vi "piezoWriteStart.vi"   [LabVIEW 2017]
uses:
  globalDevices.vi
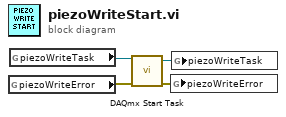
[diagram p0: block diagram]
diagram:
  n1 = global read "globalDevices.vi" "piezoWriteError"() -> (w3:errorcluster)
  n2 = global read "globalDevices.vi" "piezoWriteTask"() -> (w4:refnum<k21>)
  n3 = call <vilib>:"DAQmx Start Task.vi"("task/channels in"=w4, "error in"=w3) -> ("task out"=w2:refnum<k21>, "error out"=w1:errorcluster)  [unwired: 12 in]
  n4 = global write "globalDevices.vi" "piezoWriteError"(w1) -> ()
  n5 = global write "globalDevices.vi" "piezoWriteTask"(w2) -> ()
